vi "pid控制-静止.vi"(0 "目标p1":dbl, 1 "当前p1":dbl, 2 "kp1":dbl, 3 "ki1":dbl, 4 "kd1":dbl, 5 "目标p2":dbl, 6 "当前p2":dbl, 7 "kp2":dbl, 8 "ki2":dbl, 9 "kd2":dbl) -> (10 "输出v":dbl)   [LabVIEW 2022 SP3]
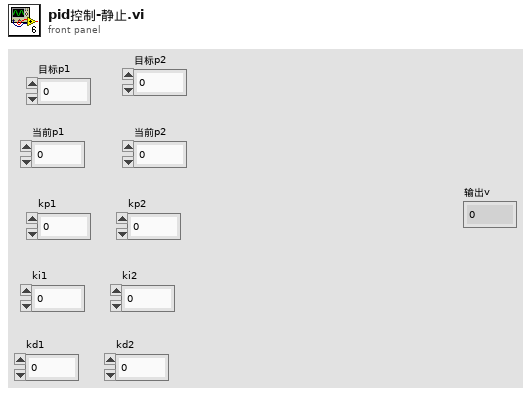
[diagram p1: front panel]
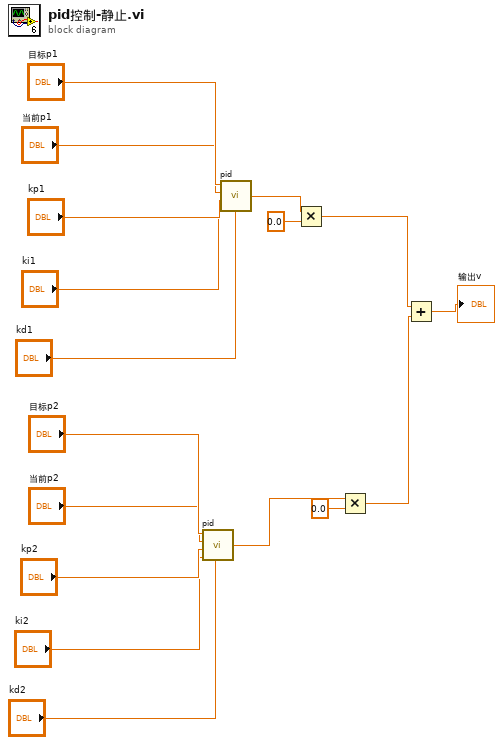
[diagram p0: block diagram]
diagram:
  n1 = call "pid.vi"("目标"="目标p2", "当前"="当前p2", "kp"="kp2", "ki"="ki2", "kd"="kd2") -> ("out"=w5:dbl)
  n2 = call "pid.vi"("目标"="目标p1", "当前"="当前p1", "kp"="kp1", "ki"="ki1", "kd"="kd1") -> ("out"=w7:dbl)
  n3 = Multiply(x=w7, y=0.0) -> (x*y=w3:dbl)
  n4 = Multiply(x=w5, y=0.0) -> (x*y=w2:dbl)
  n5 = Add(x=w3, y=w2) -> (x+y=→"输出v":dbl)
